vi "Chroma 1905x Series Configure Hipot ARC Limit.vi"(7 "Mode":T1 items=["AC", "DC"], 8 "error in (no error)":errorcluster, 9 "ARC Limit [A]":dbl min=0.0 format="%_4p", 10 "Step":T2=1 min=1 max=99 step=1, 11 "VISA resource name":refnum<visa-resource-name>) -> (0 "error out":errorcluster, 3 "VISA resource name out":refnum<visa-resource-name>)   [LabVIEW 2025]
uses:
  Type Def/steps--ring.ctl
  Type Def/AC-DC modes--ring.ctl
panel:
  # "Configure ARC Limit"
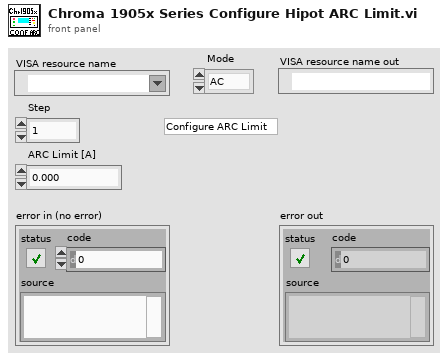
[diagram p1: front panel]
types:
  T1 = typedef "AC-DC modes--ring.ctl" = i32
  T2 = typedef "steps--ring.ctl" = u8
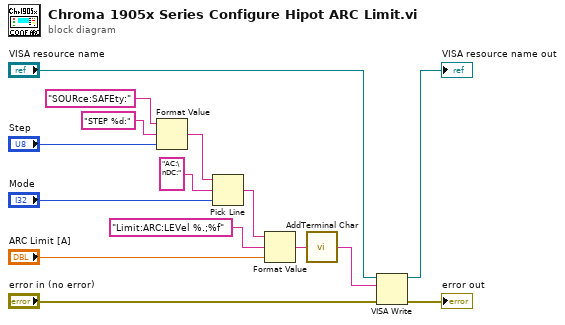
[diagram p0: block diagram]
diagram:
  n1 = Format Value(string ("")="SOURce:SAFEty:", format string="STEP %d:", value (0)="Step") -> (output string=w12:string)
  n2 = Pick Line(string ("")=w12, multi-line string="AC:\nDC:", line index="Mode") -> (output string=w10:string)
  n3 = Format Value(string ("")=w10, format string="Limit:ARC:LEVel %.;%f", value (0)="ARC Limit [A]") -> (output string=w2:string)
  n4 = call "AddTerminal Char.vi"("Cmd string"=w2) -> ("Concatenated String"=w1:string)  [unwired: 4 in]
  n5 = VISA Write(VISA resource name="VISA resource name", write buffer=w1, error in (no error)="error in (no error)") -> (VISA resource name out=→"VISA resource name out":refnum<visa-resource-name>, error out=→"error out":errorcluster)  [unwired: 1 out]
